vi "Remove Cluster & Tab Refs.vi"(8 "Error In":errorcluster, 11 "VI Refnum In":refnum<vi>) -> (0 "error out":errorcluster, 2 "Refs Out":refnum<vi>[](array[refnum]), 3 "VI Refnum Out":refnum<vi>)   [LabVIEW 2011]
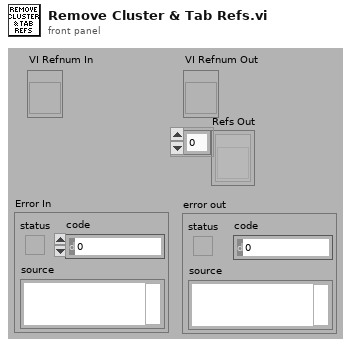
[diagram p1: front panel]
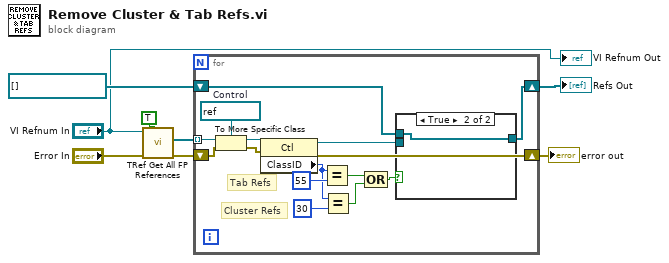
[diagram p0: block diagram]
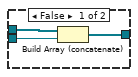
[diagram p2: hidden frame]
diagram:
  n1 = call <vilib>:"TRef Get All FP References.vi"("Ignore Decorations?"=TRUE, "error in (no error)"="Error In", "VI Refnum"="VI Refnum In") -> ("error out"=w6:errorcluster, "All FP Objects"=w7:refnum<vi>[])  [unwired: 4 in, 3 out]
  n2 = for {
    tunnel: w7 -> [w15] mode=indexing
    shift-right: [w12] -> w2
    shift-left: w6 -> [w14]
    shift-right: [w10] -> w4
    shift-left: refnum<vi>[] [] -> [w11]
    w9 = refnum<vi> refnum  # Control
    # "Cluster Refs"
    # "Tab Refs"
    n3 = To More Specific Class(target class=w9, reference=w15, error in=w14) -> (specific class reference=w18:refnum<vi>, error out=w17:errorcluster)
    n4 = property class="Ctl"(reference=w18, error in=w17) -> (reference out=w13:refnum<vi>, error out=w12:errorcluster, "ClassID"=w19:u32)
    n5 = Equal?(x=w19, y=u32 55) -> (x = y?=w22:bool)
    n6 = Equal?(x=w19, y=u32 30) -> (x = y?=w23:bool)
    n7 = Compound Arithmetic op=OR(w22, w23) -> (w16:bool)
    n8 = case shown="True" w16 {
      tunnel: w13 -> [w26 _]
      tunnel: [w25 w27] -> w10
      tunnel: w11 -> [w24 w27]
      frame False {
        n9 = Build Array (concatenate)(w24, w26) -> (w25:refnum<vi>[])
      }
      frame True {
      }
    }
  }
  "Refs Out" <- w4
  "error out" <- w2
  "VI Refnum Out" <- "VI Refnum In"
